vi "Get Path Regex.vi"(8 "error in (no error)":errorcluster, 11 "File Upload Controller in":refnum<class "File Upload Controller.lvclass">) -> (0 "error out":errorcluster, 2 "Path Regex":string, 3 "File Upload Controller out":refnum<class "File Upload Controller.lvclass">)   [LabVIEW 2020, in "File Upload Controller.lvclass"]
uses:
  File Upload Controller.lvclass
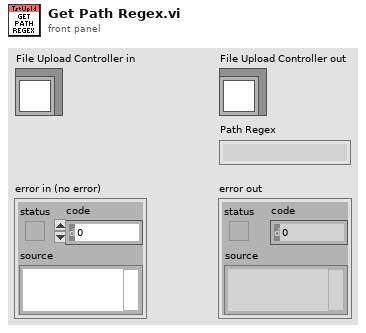
[diagram p1: front panel]
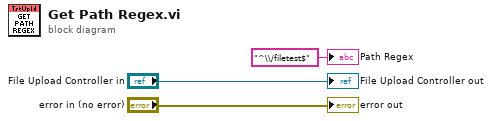
[diagram p0: block diagram]
diagram:
  "error out" <- "error in (no error)"
  "File Upload Controller out" <- "File Upload Controller in"
  "Path Regex" <- "^\\/filetest$" ("Path Regex")
